vi "Set Wavelength.vi"(8 "error in (no error)":errorcluster, 10 "Wavelength":dbl, 11 "Simulated-Topas in":refnum<class "Simulated-Topas.lvclass">) -> (0 "error out":errorcluster, 3 "Simulated-Topas out":refnum<class "Simulated-Topas.lvclass">)   [LabVIEW 2019, in "Simulated-Topas.lvclass"]
uses:
  Simulated-Topas.lvclass
  Simulated-Topas.lvclass/Simulated-Topas.ctl
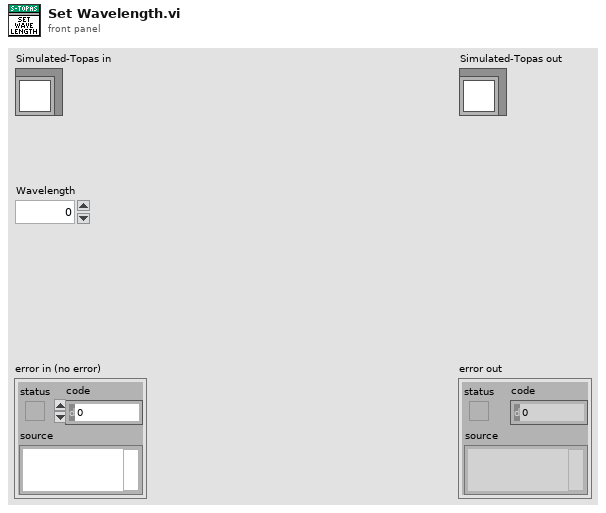
[diagram p1: front panel]
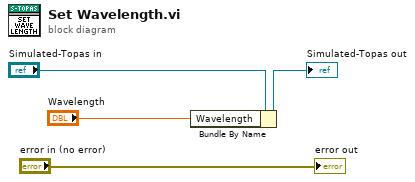
[diagram p0: block diagram]
diagram:
  n1 = Bundle By Name(cluster="Simulated-Topas in", "Wavelength"="Wavelength") -> (→"Simulated-Topas out":refnum<class "Simulated-Topas.lvclass">)
  "error out" <- "error in (no error)"
